vi "THz Time(SR830_VC)_Delay_LGS.vi"(1 "ESP300 Axis1":i8=1, 2 "ESP300 Address1":string="1", 4 "Lockin Address":string="12") -> ()   [LabVIEW 2010]
uses:
  <vilib>/Utility/file.llb/Write To Spreadsheet File (DBL).vi
panel:
  out "Boolean 2":bool
  in  "Position 3":sgl=3.4 format="%#.4f"
  in  "Set Position 2":bool
  out "error out":errorcluster
  out "Position 2":dbl[](array[numeric])=[2.395] format="%.6f"
  in  "error in":errorcluster
  out "Running":bool caption="Mercury_GCS_Configuration_Setup.vi is running"
  out "Conn. Axis":string[](array[string])=["1"]
  out "Identification":string="(c)2013 Physik Instrumente(PI) Karlsruhe, C-863.11,0,1.3.0.7"
  in  "SaveFile name":string="t"
  in  "Interdelay (ms)":dbl=10.0
  in  "pre delay(ms)":dbl=100.0
  out "Current deceleration":dbl=100.0
  in  "Acceleration":dbl
  out "Current acceleration":dbl=100.0
  in  "Set Acc":bool
  out "Current Velocity":dbl=25.0
  in  "Delay1 Stage":dbl
  in  "Set Velocity":bool
  in  "Reset Range":bool
  out "Boolean":bool
  out "MinValue":dbl format="%#.3p"
  out "MinPosition":dbl format="%#.3f"
  out "Lock-in Y-Channel":dbl=-7.0941e-11 format="%#.3p"
  out "Lock-in X-Channel":dbl=5.62071e-10 format="%#.3p"
  out "THz Time-domain Signal Wave":cluster{"x-axis":sgl[], "y-axis":dbl[]}(graph)={"x-axis"=[3.4, 3.395, 3.39, 3.385, 3.38, 3.375, 3.3700001, 3.365, 3.3600001, 3.355, 3.3500001, 3.345, 3.3400002, 3.335, 3.3300002, 3.325, 3.3200002, 3.315, 3.3100002, 3.305, 3.3000002, 3.295, 3.2900002, 3.285, 3.2800002, 3.275, 3.27, 3.265, 3.26, 3.255, 3.25, 3.2450001, 3.24, 3.2350001, 3.23, 3.2250001, 3.22, 3.2150002, 3.21, 3.2050002, 3.2, 3.1950002, 3.19, 3.1850002, 3.18, 3.1750002, 3.17, 3.1650002, 3.16, 3.1550002, 3.15, 3.1450002, 3.14, 3.135, 3.13, 3.125, 3.1200001, 3.115, 3.1100001, 3.105, 3.1000001, 3.095, 3.0900002, 3.085, 3.0800002, 3.075, 3.0700002, 3.065, 3.0600002, 3.055, 3.0500002, 3.045, 3.0400002, 3.035, 3.0300002, 3.025, 3.0200002, 3.015, 3.01, 3.005, 3.0, 2.9950001, 2.99, 2.9850001, 2.98, 2.9750001, 2.97, 2.9650002, 2.96, 2.9550002, 2.95, 2.9450002, 2.94, 2.9350002, 2.93, 2.9250002, 2.92, 2.9150002, 2.91, 2.9050002, 2.9, 2.8950002, 2.89, 2.885, 2.88, 2.875, 2.8700001, 2.865, 2.8600001, 2.855, 2.8500001, 2.845, 2.8400002, 2.835, 2.8300002, 2.825, 2.8200002, 2.815, 2.8100002, 2.805, 2.8000002, 2.795, 2.7900002, 2.785, 2.7800002, 2.775, 2.7700002, 2.765, 2.7600002, 2.755, 2.75, 2.7450001, 2.74, 2.7350001, 2.73, 2.7250001, 2.72, 2.7150002, 2.71, 2.7050002, 2.7, 2.6950002, 2.69, 2.6850002, 2.68, 2.6750002, 2.67, 2.6650002, 2.66, 2.6550002, 2.65, 2.6450002, 2.64, 2.6350002, 2.63, 2.625, 2.6200001, 2.615, 2.6100001, 2.605, 2.6000001, 2.595, 2.5900002, 2.585, 2.5800002, 2.575, 2.5700002, 2.565, 2.5600002, 2.555, 2.5500002, 2.545, 2.5400002, 2.535, 2.5300002, 2.525, 2.5200002, 2.515, 2.5100002, 2.505, 2.5, 2.4950001, 2.49, 2.4850001, 2.48, 2.4750001, 2.47, 2.4650002, 2.46, 2.4550002, 2.45, 2.4450002, 2.44, 2.4350002, 2.43, 2.4250002, 2.42, 2.4150002, 2.41, 2.4050002, 2.4, 2.3950002], "y-axis"=array[202 elements]}
  in  "Autosave Directory for Long-term Average Scan":path=path "D:/Soon/140901_delay_test/2_VC_delay_ESP_-2.35/1_VC_delay"
  out "Phase":cluster{"f0":dbl, "df":dbl, "magnitude":dbl[]}(graph)={"f0"=0.0, "df"=0.14851486070616432, "magnitude"=[3.141592653589793, -1.1082186029585688, 2.1245945726281503, -0.5802126962218755, 2.9522431871923738, 0.25355132108658424, -2.5001587400129117, 1.0450360548561866, -1.6833529420673685, 1.9054335161918228, -0.7535788037728205, 2.8437560114605995, 0.1867891479959547, -2.5687719161866958, 1.0293610676943812, -1.7670984731304367, 1.7396136198319216, -0.989399029539729, 2.5333749473756697, 0.8404425122915157, -3.0418476408700195, 1.801491493426078, 1.2291977401939342, 2.193306480389313, 1.1536290801184514, 2.257021637212434, 1.4812870523644348, 2.188959750025471, 1.966995842051201, 1.8991000587928113, 2.316846473675966, 1.7957148476473666, 2.343784775169297, 2.055723593650246, 1.8995404855444666, 2.3374703620389807, 1.7334801576564551, 2.5115455204750092, 1.9597467730439078, 2.2954790599099035, 2.198181356679205, 2.1422497310116677, 2.228848712078954, 2.3604901133382894, 1.9776993845037527, 2.602909416876564, 2.0799347375491797, 2.4419998834544696, 2.3534588247198736, 2.2439655455562337, 2.367780240538884, 2.4173118073649276, 2.13794690411644, 2.6001847828499938, 2.2538070428436865, 2.4392433056261886, 2.5322980937687722, 2.33220876018927, 2.5581206126688922, 2.4920111361083035, 2.365959844925607, 2.6396344462612515, 2.387346853088604, 2.663819735565773, 2.503292776172557, 2.6066427525464575, 2.596199386556665, 2.5917147401712675, 2.5966251179974464, 2.6741740931066458, 2.575163618331821, 2.758796254024769, 2.606630146141833, 2.698588779947026, 2.779755754618168, 2.636241327225838, 2.859969608313545, 2.68829051279584, 2.7969939565985547, 2.795740014252736, 2.7620236189146024, 2.857190149539915, 2.8576368807511114, 2.7988186860636706, 2.9527385937994426, 2.8126212545415386, 2.9271634690601185, 2.96078760907565, 2.7401621755492296, -3.0621438857467163, 2.5801858239187037, -2.741093203572613, 2.771636401079869, -2.8921243601658513, -3.091948951572802, 1.9572111607568423, -2.7375815827125485, 2.554987619803606, -2.850283932292324, 3.0341936848447073, 3.139143526249259]}
  out "elapsed time":string=" 0 h  12 m  48 s"
  in  "OK Button":bool
  out "Data Type":string="outp ? 1"
  in  "Enum":enum16{"X", "Y", "Abs"}(ring)
  out "MaxValue":dbl format="%#.3p"
  out "MaxPosition":dbl format="%#.3f"
  in  "Position":sgl format="%#.4f"
  in  "Find Max":bool
  in  "Set Position":bool
  in  "Save Data":bool
  in  "SCAN":bool
  in  "Exit Program":bool
  out "Amplitude":cluster{"f0":dbl, "df":dbl, "magnitude":dbl[]}(graph)={"f0"=0.0, "df"=0.14851486070616432, "magnitude"=[3.52573264851484e-11, 8.389855621430922e-10, 2.225761799960767e-09, 3.4042126658161336e-09, 4.230842896022254e-09, 4.467306313802578e-09, 4.228754619739681e-09, 3.6175759039566052e-09, 2.7932538533113405e-09, 2.0909677390642694e-09, 1.4830038497464771e-09, 1.0735909873360868e-09, 7.513836201453385e-10, 5.085801170819804e-10, 3.409708772444367e-10, 2.0157630953836574e-10, 1.3092497815900202e-10, 5.049635088240611e-11, 3.21982450563289e-11, 1.6834701069452993e-11, 7.165882992001707e-12, 1.3534244019293799e-11, 2.2560794068677396e-12, 1.0955642605171567e-11, 3.936119948051029e-12, 9.190533457493373e-12, 4.4193088993100694e-12, 6.762265647261314e-12, 4.993312878347624e-12, 5.062736813562155e-12, 5.24252743088094e-12, 5.787564208573698e-12, 3.5338798468168525e-12, 6.289625941575823e-12, 2.9009219878310403e-12, 5.735399147740872e-12, 4.098798711026944e-12, 4.0941543980206186e-12, 5.005680034820198e-12, 2.9952585898831173e-12, 4.635819232904141e-12, 3.483558839132468e-12, 3.5438954539821336e-12, 4.019219618061033e-12, 3.530627852632409e-12, 3.4790764329431817e-12, 4.215077525071282e-12, 2.6292492576384014e-12, 3.696721717997553e-12, 3.400423534031585e-12, 2.5887642494668405e-12, 3.943756030791582e-12, 2.5289746794441754e-12, 3.401204539630353e-12, 3.10293276186898e-12, 2.786775807858238e-12, 2.9186601113132677e-12, 3.284595365146064e-12, 2.271033822874899e-12, 3.5054000253471667e-12, 2.2657565242544363e-12, 3.112172318680258e-12, 2.6330104473143568e-12, 2.7634443891954928e-12, 2.7484453359122282e-12, 2.592035676554931e-12, 2.5633028950781254e-12, 2.6521106649509693e-12, 2.360345428093699e-12, 2.7497689895804224e-12, 2.3635944544452143e-12, 2.5866385290965327e-12, 2.5442012769231896e-12, 2.298983787328914e-12, 2.624194910906667e-12, 2.384593975973384e-12, 2.3523429224266368e-12, 2.5577359065613025e-12, 2.221370415250699e-12, 2.4629634177599407e-12, 2.3284037072725584e-12, 2.2392891386041413e-12, 2.4830764922560122e-12, 2.1850697748689936e-12, 2.3325327936824436e-12, 2.4734800041535514e-12, 2.041958899932065e-12, 2.6672550572923e-12, 1.847654298403158e-12, 2.668652435775197e-12, 2.456539312232025e-12, 1.9162881391774236e-12, 3.5876527691091694e-12, 5.308809354301319e-13, 4.197872609875915e-12, 1.5590595736913964e-12, 3.349567160539913e-12, 2.5611964195912033e-12, 2.0676305856675026e-12, 2.350754443680646e-12, 2.2948601507955558e-12]}
  in  "Short term \nAverage#":i8=2
  out "Numeric 2":i8=15
  in  "Long term Average#":dbl=16.0
  in  "Step":sgl=0.005 min=0 max=10000 format="%.3f"
  in  "End Postion":sgl=2.4 min=-400 max=400 format="%#.3f"
  in  "Start Position":sgl=3.4 min=-400 max=400 format="%#.3f"
  # "This Program Run First (1) and then Run the Approach Program (2)"
  # "THz Experiment"
  # "``"
  # "Auto-offset"
  # "Input Data"
  # "Delay Line (VC)"
  # "Point Avg"
  # "Long Avg"
  # "Turn Number"
  # "mm"
  # "mm"
  # "MAX"
  # "MIN"
  # "other step\nposition"
  # "stage \nposition"
  # "stage \nposition"
  # "value"
  # "value"
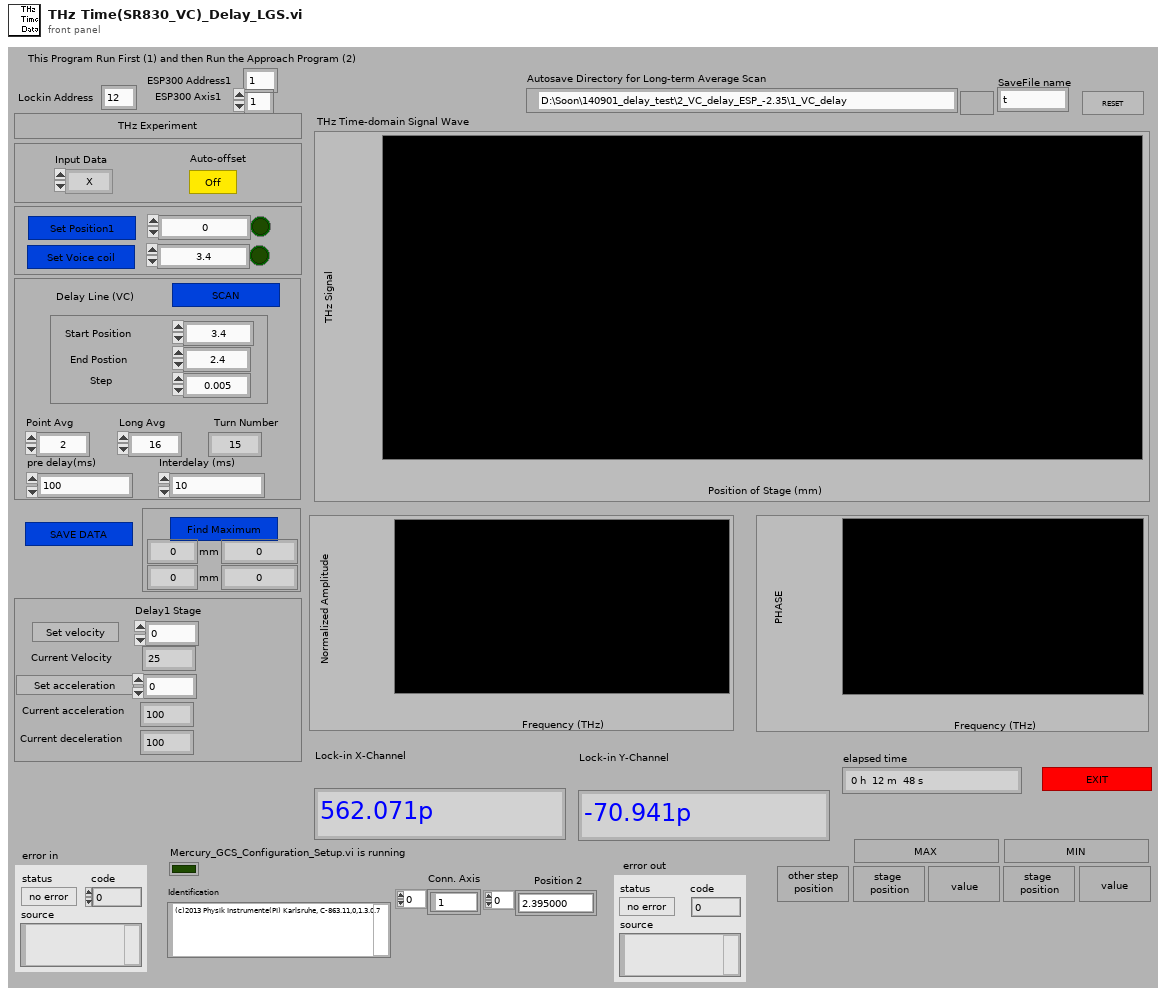
[diagram p1: front panel]
types:
  T1 = cluster{"System no.":i32, "error out":errorcluster}
  T2 = cluster{"Step Number":i32, "Step":sgl, "Start Position":sgl, "Time-out":i32, "Lockin Address":string, "Short term \nAverage#":i8, "System no.":i32, "error out":errorcluster, "Value":string, "pre delay(ms)":dbl, "Interdelay (ms)":dbl, "Autosave Directory for Long-term Average Scan":path}
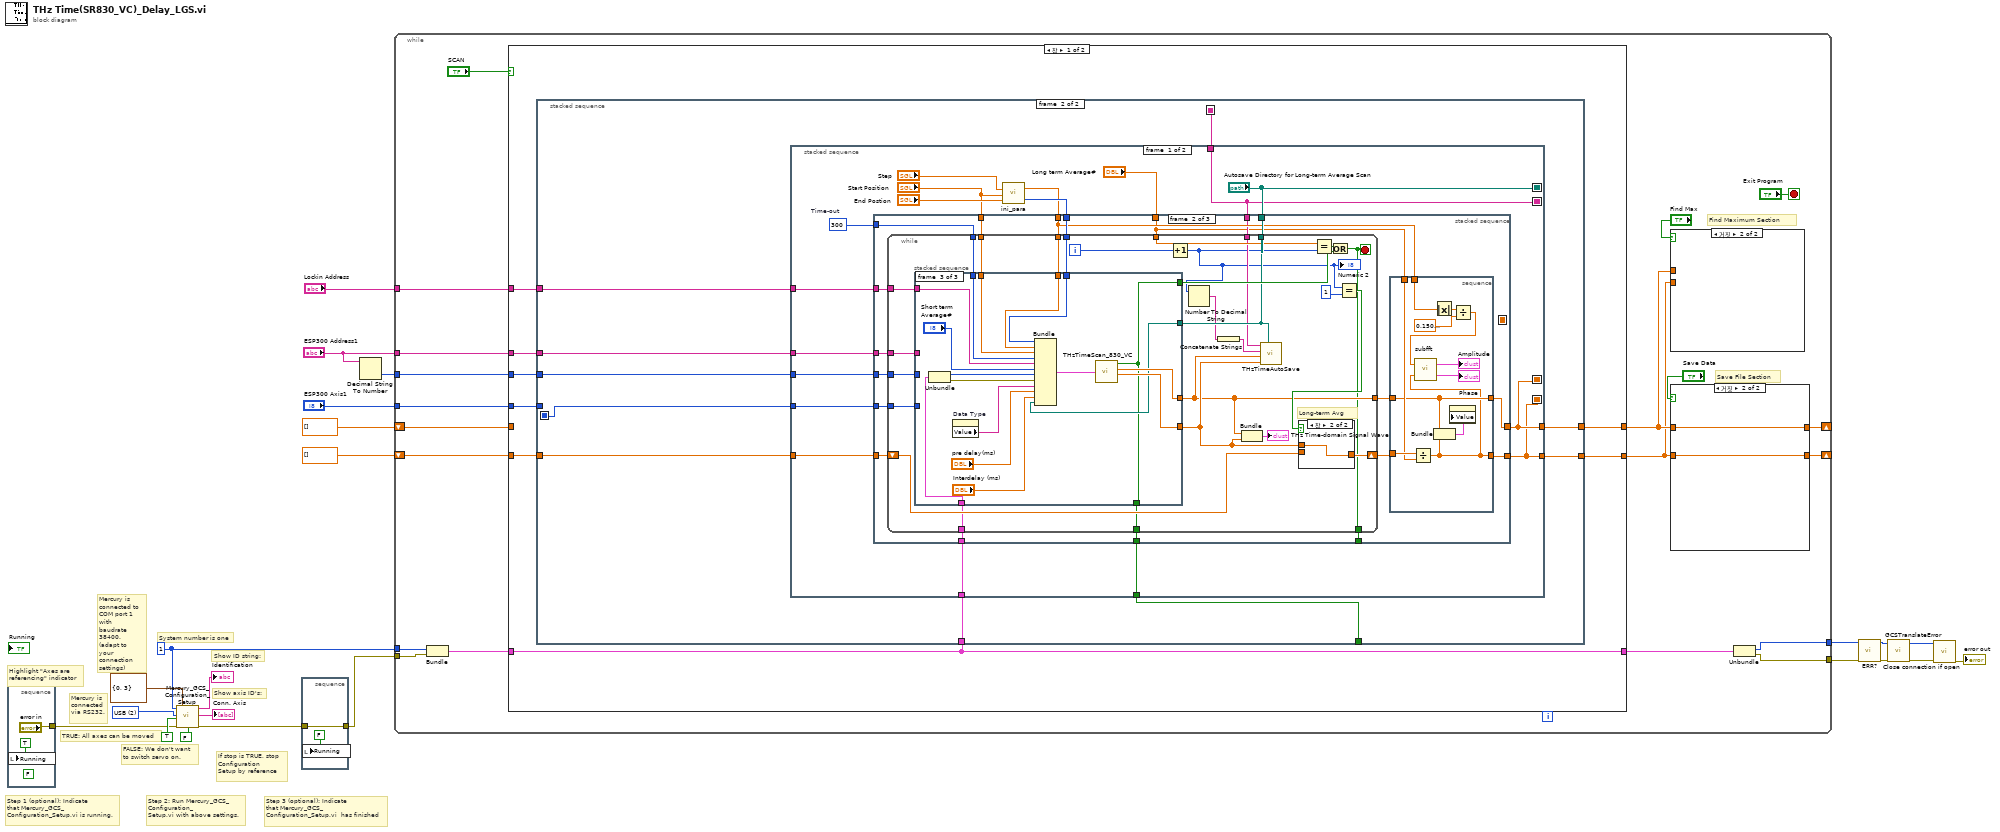
[diagram p0: block diagram]
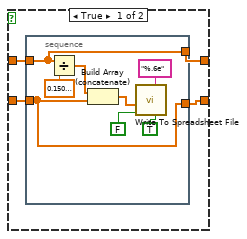
[diagram p2: hidden frame]
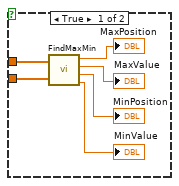
[diagram p3: hidden frame]
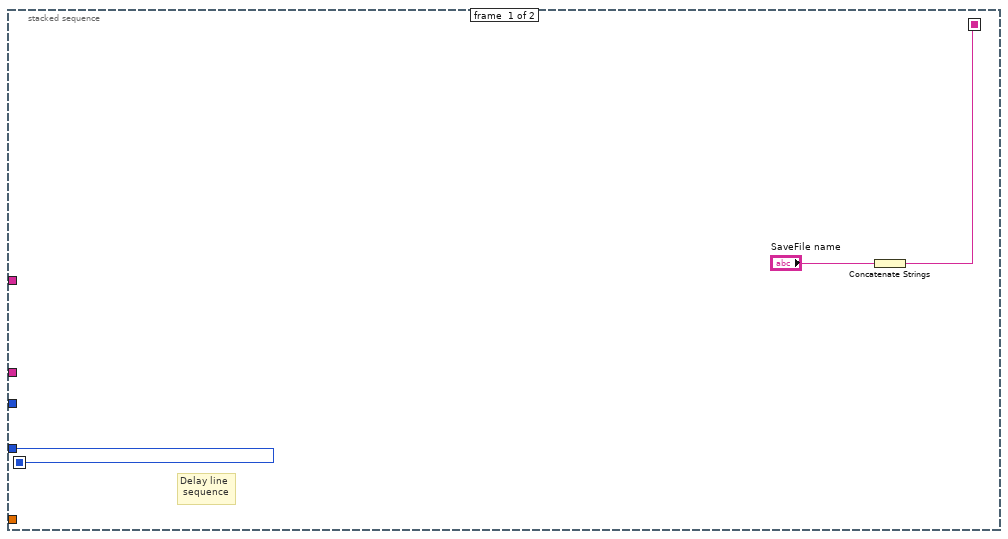
[diagram p4: hidden frame]
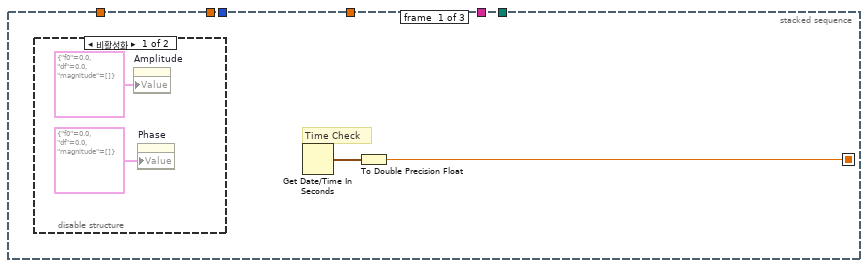
[diagram p5: hidden frame]
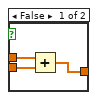
[diagram p7: hidden frame]
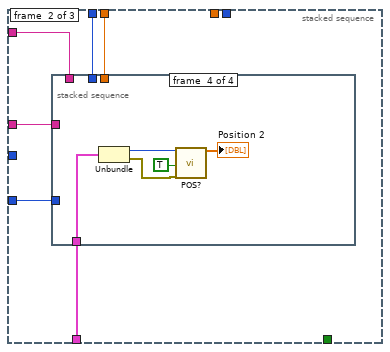
[diagram p9: hidden frame]
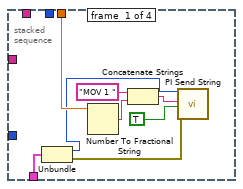
[diagram p10: hidden frame]
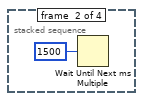
[diagram p11: hidden frame]
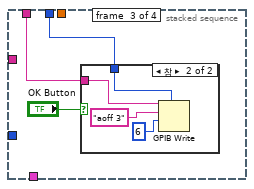
[diagram p12: hidden frame]
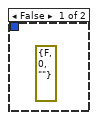
[diagram p13: hidden frame]
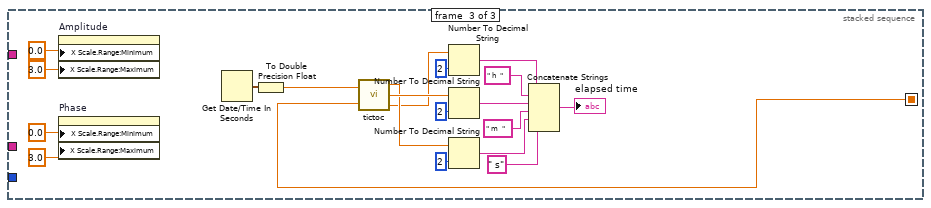
[diagram p14: hidden frame]
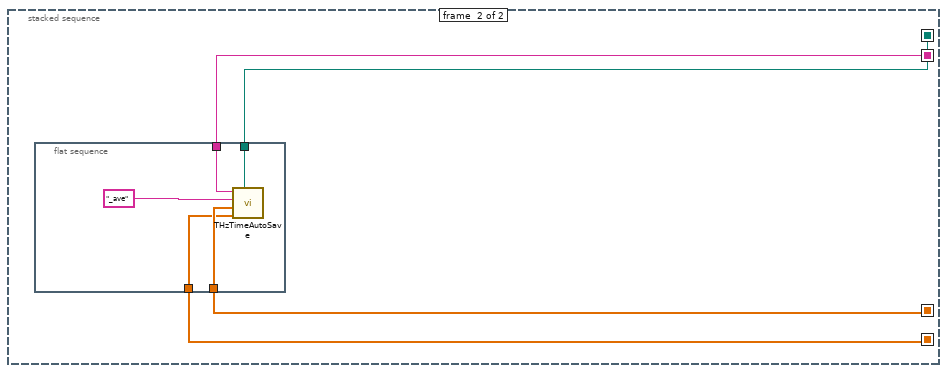
[diagram p15: hidden frame]
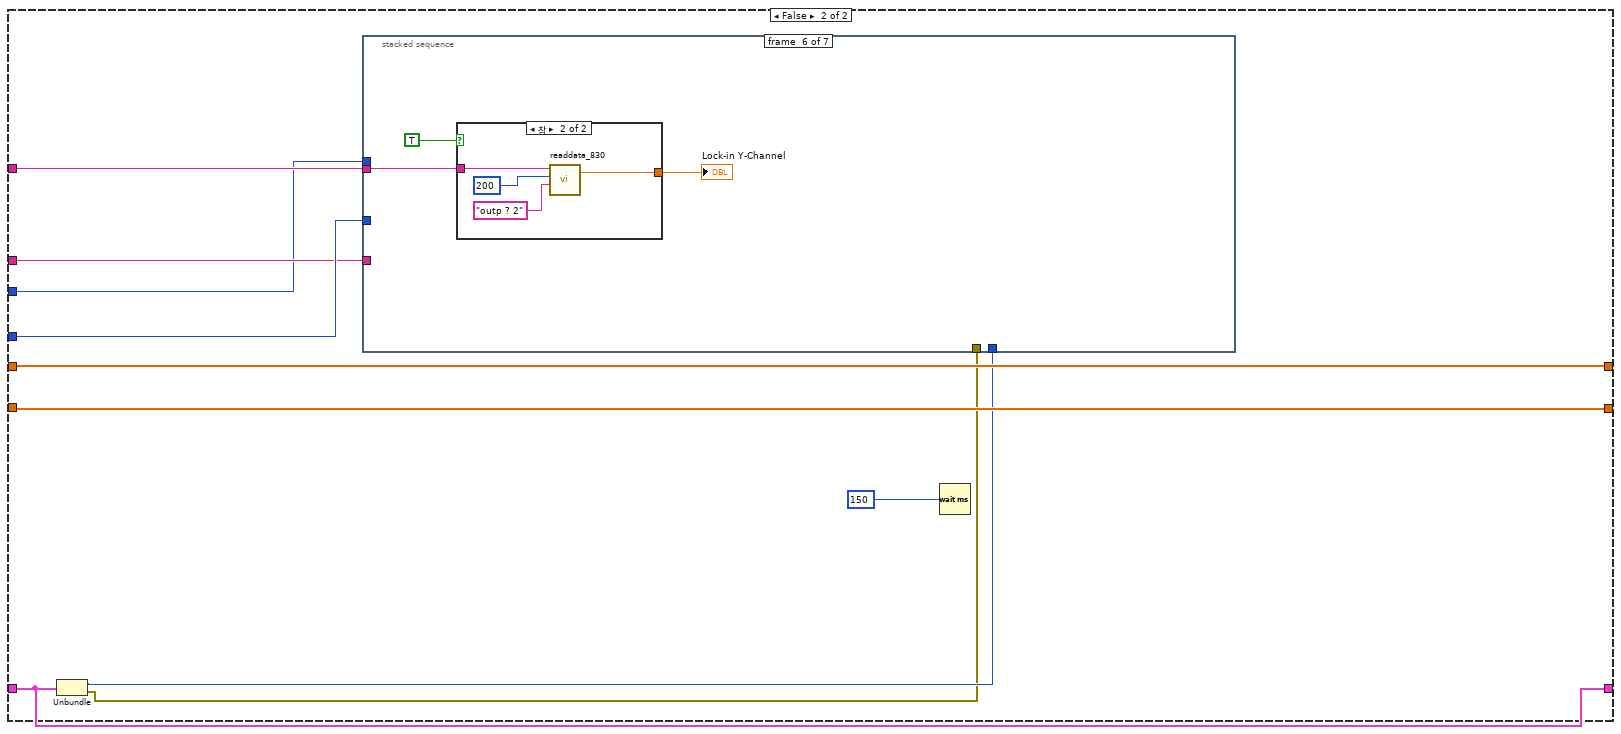
[diagram p16: hidden frame]
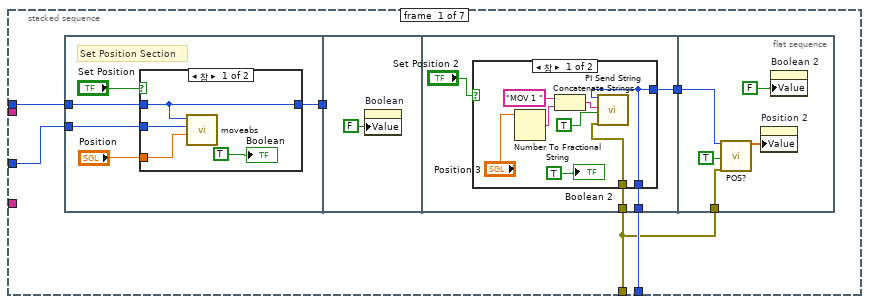
[diagram p17: hidden frame]
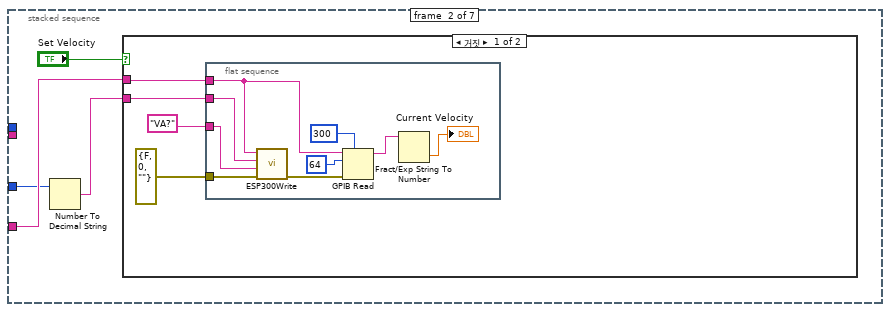
[diagram p20: hidden frame]
diagram:
  w8 = u16 2 items=["RS232", "RS232 DaisyChain", "USB", "USB_DaisyChain"] ("Interface")
  w7 = 1 ("System no.")
  # "Mercury is\nconnected\nvia RS232."
  # "If stop is TRUE, stop \nConfiguration\nSetup by reference"
  # "Mercury is\nconnected to\nCOM port 1\nwith baudrate\n38400.\n(adapt to your\nconnection\nsettings)"
  # "Step 3 (optional): Indicate\nthat Mercury_GCS_\nConfiguration_Setup.vi  has finished"
  # "Step 2: Run Mercury_GCS_\nConfiguration_\nSetup.vi with above settings."
  # "Step 1 (optional): Indicate\nthat Mercury_GCS_\nConfiguration_Setup.vi is running."
  # "Highlight \"Axes are\nreferencing\" indicator"
  # "Show axis ID's:"
  # "Show ID string:"
  # "FALSE: We don't want\nto switch servo on."
  # "TRUE: All axes can be moved"
  # "System number is one"
  n1 = stacked-sequence {
    tunnel: ["error in"] -> w11
    frame #0 {
      (unwired) FALSE ("stop")
      n2 = local write "Running"(TRUE ("Running")) -> ()
    }
  }
  n3 = call "Mercury_GCS_Configuration_Setup.vi"("System no."=w7, "Interface"=w8, "All axes?"=TRUE, "error in"=w11, "RS232 settings"=cluster{"RS232 Portnumber":i32, "Baudrate":u16} {"RS232 Portnumber"=0, "Baudrate"=3}, "Switch servo on?"=FALSE ("Use dialog to define\nconnected stages?")) -> ("Identification"=→"Identification":string, "Conn. \nAxes"=→"Conn. Axis":string[], "error out"=w12:errorcluster)  [unwired: 7 in, 4 out]
  n4 = stacked-sequence {
    tunnel: w12 -> [w25]
    tunnel: [w25] -> w6
    frame #0 {
      n5 = local write "Running"(FALSE ("Running")) -> ()
    }
  }
  n6 = Decimal String To Number(string="ESP300 Address1") -> (number=w16:i32)  [unwired: 2 in, 1 out]
  n7 = while {
    tunnel: "ESP300 Axis1" -> [w41]
    tunnel: "Lockin Address" -> [w33]
    shift-right: [w38] -> _
    shift-left: sgl[] [] -> [w40]
    shift-right: [w37] -> _
    shift-left: dbl[] [] -> [w39]
    tunnel: "ESP300 Address1" -> [w34]
    tunnel: w16 -> [w32]
    tunnel: w7 -> [w31]
    tunnel: w6 -> [w30]
    tunnel: [w27] -> w2
    tunnel: [w26] -> w1
    stop <- "Exit Program" stop-if-true
    # "Save File Section"
    # "Find Maximum Section"
    n8 = Bundle("System no."=w31, "error out"=w30) -> (w29:T1)  [unwired: 1 in]
    n9 = case shown="참" "SCAN" {
      tunnel: w41 -> [w73 w252]
      tunnel: [w72 w249] -> w36
      tunnel: [w71 w248] -> w35
      tunnel: w40 -> [_ w249]
      tunnel: w39 -> [w70 w248]
      tunnel: w34 -> [w69 w250]
      tunnel: w33 -> [w68 w247]
      tunnel: w32 -> [w67 w246]
      tunnel: w29 -> [w66 w243]
      tunnel: [w66 w243] -> w28
      frame True {
        n10 = stacked-sequence {
          seq-local: [w76 _] -> [_ w79]
          seq-local: [w74 _] -> [_ w80]
          tunnel: w73 -> [w76 _]
          tunnel: [_ w86] -> w72
          tunnel: [_ w85] -> w71
          tunnel: w70 -> [_ w84]
          tunnel: w69 -> [_ w83]
          tunnel: w68 -> [_ w82]
          tunnel: w67 -> [_ w81]
          tunnel: [_ w77] -> _
          tunnel: w66 -> [_ w78]
          frame #0 {
            # "Delay line\n sequence"
            n11 = Concatenate Strings("SaveFile name") -> (w74:string)
          }
          frame #1 {
            n12 = stacked-sequence {
              seq-local: [w94 _] -> [_ w235]
              seq-local: [w93 _] -> [_ w234]
              seq-local: ["Autosave Directory for Long-term Average Scan" _] -> [_ w236]
              seq-local: [w89 _] -> [_ w237]
              tunnel: w79 -> [w104 _]
              tunnel: [w94 _] -> w86
              tunnel: [w93 _] -> w85
              tunnel: w84 -> [w97 _]
              tunnel: w83 -> [w96 _]
              tunnel: [w95 _] -> w77
              tunnel: w82 -> [w91 _]
              tunnel: w81 -> [w90 _]
              tunnel: w80 -> [w89 _]
              tunnel: w78 -> [w87 _]
              frame #0 {
                w103 = 300  # Time-out
                n13 = call "ini_para.vi"("End Position"="End Postion", "Start Position"="Start Position", "Step"="Step") -> ("Step Number"=w100:i32, "Step"=w99:sgl)
                n14 = stacked-sequence {
                  seq-local: [w105 _ _] -> [_ _ w214]
                  tunnel: w103 -> [_ w127 _]
                  tunnel: "Long term Average#" -> [_ w110 _]
                  tunnel: w104 -> [_ w126 _]
                  tunnel: w100 -> [_ w124 _]
                  tunnel: w99 -> [_ w122 _]
                  tunnel: "Start Position" -> [_ w125 _]
                  tunnel: "Autosave Directory for Long-term Average Scan" -> [_ w123 _]
                  tunnel: [_ w113 _] -> w94
                  tunnel: [_ w121 _] -> w93
                  tunnel: w97 -> [_ w119 _]
                  tunnel: w96 -> [_ w120 _]
                  tunnel: w89 -> [_ w118 _]
                  tunnel: [_ w117 _] -> w95
                  tunnel: w91 -> [_ w116 _]
                  tunnel: w90 -> [_ w115 _]
                  tunnel: [_ w111 _] -> _
                  tunnel: w87 -> [_ w109 _]
                  frame #0 {
                    # "Time Check"
                    n15 = disable-structure shown="비활성화" {
                      frame Disabled {
                        n16 = property on="Amplitude" class="WFGraph (엄격한)"("Value"=cluster{"f0":dbl, "df":dbl, "magnitude":dbl[]} {"f0"=0.0, "df"=0.0, "magnitude"=[]} ("Spectrum")) -> ()  [unwired: 2 in, 2 out]
                        n17 = property on="Phase" class="WFGraph (엄격한)"("Value"=cluster{"f0":dbl, "df":dbl, "magnitude":dbl[]} {"f0"=0.0, "df"=0.0, "magnitude"=[]} ("Spectrum")) -> ()  [unwired: 2 in, 2 out]
                      }
                      frame Enabled {
                      }
                    }
                    n18 = Get Date/Time In Seconds() -> (seconds since 1Jan1904=w106:timestamp)
                    n19 = To Double Precision Float(number=w106) -> (double precision float=w105:dbl)
                  }
                  frame #1 {
                    n20 = while {
                      tunnel: w110 -> [w164]
                      tunnel: w127 -> [w165]
                      tunnel: w126 -> [w161]
                      tunnel: w125 -> [w160]
                      tunnel: w122 -> [w159]
                      tunnel: w124 -> [w158]
                      tunnel: w123 -> [w153]
                      shift-right: [w144] -> w112
                      shift-left: w119 -> [w156]
                      tunnel: [w146] -> w114
                      tunnel: w120 -> [w155]
                      tunnel: w118 -> [w152]
                      tunnel: [w154] -> w117
                      tunnel: w116 -> [w149]
                      tunnel: w115 -> [w148]
                      tunnel: [w143] -> w111
                      tunnel: w109 -> [w141]
                      i -> [w140]
                      stop <- w143 stop-if-true
                      # "Long-term Avg"
                      n21 = stacked-sequence {
                        tunnel: w165 -> [_ w175 w212]
                        tunnel: [_ _ w204] -> w162
                        tunnel: w161 -> [_ w174 _]
                        tunnel: w160 -> [_ w173 w200]
                        tunnel: w159 -> [_ _ w201]
                        tunnel: w158 -> [_ _ w213]
                        tunnel: [_ _ w209] -> w146
                        tunnel: [_ _ w208] -> w150
                        tunnel: w155 -> [_ w172 _]
                        tunnel: w153 -> [_ _ w205]
                        tunnel: [_ _ w204] -> w154
                        tunnel: w149 -> [_ w171 w203]
                        tunnel: w148 -> [_ _ _]
                        tunnel: w141 -> [_ w170 w199]
                        frame #0 {
                        }
                        frame #1 {
                          n22 = stacked-sequence {
                            tunnel: w175 -> [_ _ w186 _]
                            tunnel: w174 -> [_ _ _ _]
                            tunnel: w173 -> [w179 _ _ _]
                            tunnel: w172 -> [_ _ _ _]
                            tunnel: w171 -> [_ _ w185 _]
                            tunnel: w170 -> [w178 _ _ w194]
                            frame #0 {
                              n23 = Unbundle(w178) -> ("System no."=w176:i32, "error out"=w177:errorcluster)
                              n24 = Number To Fractional String(number=w179) -> (F-format string=w180:string)  [unwired: 3 in]
                              n25 = Concatenate Strings("MOV 1 ", w180) -> (w183:string)
                              n26 = call "PI Send String.vi"("System no."=w176, "String to send"=w183, "Attach termination char.?"=TRUE ("Attach Linefeed?"), "error in"=w177) -> ()  [unwired: 15 in, 1 out]
                            }
                            frame #1 {
                              n27 = Wait Until Next ms Multiple(millisecond multiple=1500) -> ()  [unwired: 1 out]
                            }
                            frame #2 {
                              n28 = case shown="참" "OK Button" {
                                tunnel: w186 -> [_ w190]
                                tunnel: w185 -> [_ w188]
                                frame False {
                                (unwired) errorcluster {"status"=FALSE, "code"=0, "source"=""} ("error in")
                                }
                                frame True {
                                n29 = GPIB Write(0:w188, 1:"aoff 3" ("data"), 2:i16 6 ("mode (0)"), 4:w190) -> ()  [unwired: 1 in, 2 out]
                                }
                              }
                            }
                            frame #3 {
                              n30 = Unbundle(w194) -> ("System no."=w193:i32, "error out"=w192:errorcluster)
                              n31 = call "POS?.vi"("System no."=w193, "All axes?"=TRUE, "error in"=w192) -> ("Position"=→"Position 2":dbl[])  [unwired: 15 in, 1 out]
                            }
                          }
                        }
                        frame #2 {
                          n32 = Unbundle(w199) -> ("System no."=w198:i32, "error out"=w197:errorcluster)
                          n33 = property on="Data Type" class="Str"() -> ("Value"=w210:string)  [unwired: 2 in, 2 out]
                          n34 = Bundle("Step Number"=w213, "Step"=w201, "Start Position"=w200, "Time-out"=w212, "Lockin Address"=w203, "Short term \nAverage#"="Short term \nAverage#", "System no."=w198, "error out"=w197, "Value"=w210, "pre delay(ms)"="pre delay(ms)", "Interdelay (ms)"="Interdelay (ms)", "Autosave Directory for Long-term Average Scan"=w205) -> (w202:T2)  [unwired: 1 in]
                          n35 = call "THzTimeScan_830_VC.vi"("input"=w202) -> ("loop stop"=w204:bool, "x-axis"=w209:sgl[], "y-axis"=w208:dbl[])  [unwired: 1 in]
                        }
                      }
                      n36 = Increment(x=w140) -> (x+1=w139:i32)
                      "Numeric 2" <- w139
                      n37 = Number To Decimal String(number=w139) -> (decimal integer string=w142:string)  [unwired: 1 in]
                      n38 = Concatenate Strings(w142) -> (w151:string)
                      n39 = Bundle("x-axis"=w146, "y-axis"=w150) -> (→"THz Time-domain Signal Wave":cluster{"x-axis":sgl[], "y-axis":dbl[]})  [unwired: 1 in]
                      n40 = call "THzTimeAutoSave.vi"("Autosave Directory for Long-term Average Scan"=w153, "y-axis"=w150, "x-axis"=w146, "String"=w151, "SaveFile name"=w152) -> ()  [unwired: 5 in]
                      n41 = Equal?(x=w164, y=w139) -> (x = y?=w163:bool)
                      n42 = Or(x=w163, y=w162) -> (x .or. y?=w143:bool)
                      n43 = Equal?(x=w139, y=1) -> (x = y?=w147:bool)
                      n44 = case shown="참" w147 {
                        tunnel: w156 -> [w167 _]
                        tunnel: w150 -> [w168 w169]
                        tunnel: [w166 w169] -> w144
                        frame False {
                          n45 = Add(x=w168, y=w167) -> (x+y=w166:dbl[])
                        }
                        frame True {
                        }
                      }
                    }
                    n46 = stacked-sequence {
                      tunnel: w122 -> [w133]
                      tunnel: w114 -> [w129]
                      tunnel: w112 -> [w131]
                      tunnel: [w128] -> w121
                      tunnel: w110 -> [w130]
                      tunnel: [w129] -> w113
                      frame #0 {
                        n47 = Divide(x=w131, y=w130) -> (x/y=w128:dbl[])
                        n48 = Absolute Value(x=w133) -> (abs(x)=w134:sgl)
                        n49 = Bundle("x-axis"=w129, w128) -> (w138:cluster{"x-axis":sgl[], dbl[]})  [unwired: 1 in]
                        n50 = property on="THz Time-domain Signal Wave" class="XYGraph (엄격한)"("Value"=w138) -> ()  [unwired: 2 in, 2 out]
                        n51 = Divide(x=w134, y=sgl 0.15) -> (x/y=w132:sgl)
                        n52 = call "subfft.vi"("y-signal"=w128, "time step"=w132) -> ("Phase"=→"Phase":cluster{"f0":dbl, "df":dbl, "real part":dbl[]}, "Amplitude"=→"Amplitude":cluster{"f0":dbl, "df":dbl, "real part":dbl[]})
                      }
                    }
                  }
                  frame #2 {
                    n53 = property on="Amplitude" class="WFGraph (엄격한)"("X Scale.Range:Minimum"=0.0 ("X Scale.Range:Maximum"), "X Scale.Range:Maximum"=3.0) -> ()  [unwired: 2 in, 2 out]
                    n54 = property on="Phase" class="WFGraph (엄격한)"("X Scale.Range:Minimum"=0.0, "X Scale.Range:Maximum"=3.0) -> ()  [unwired: 2 in, 2 out]
                    n55 = Get Date/Time In Seconds() -> (seconds since 1Jan1904=w219:timestamp)
                    n56 = To Double Precision Float(number=w219) -> (double precision float=w218:dbl)
                    n57 = call "tictoc.vi"("Value"=w218, "Value 2"=w214) -> ("sec"=w216:dbl, "min"=w217:dbl, "hour"=w215:dbl)
                    n58 = Number To Decimal String(number=w215, width (-)=i16 2) -> (decimal integer string=w224:string)
                    n59 = Number To Decimal String(number=w217, width (-)=i16 2) -> (decimal integer string=w230:string)
                    n60 = Number To Decimal String(number=w216, width (-)=i16 2) -> (decimal integer string=w229:string)
                    n61 = Concatenate Strings(w224, " h  " ("Substring"), w230, " m  " ("Substring"), w229, " s" ("Substring")) -> (→"elapsed time":string)
                  }
                }
              }
              frame #1 {
                n62 = flat-sequence {
                  tunnel: w236 -> [w242]
                  tunnel: w237 -> [w241]
                  tunnel: w235 -> [w240]
                  tunnel: w234 -> [w239]
                  frame #0 {
                    n63 = call "THzTimeAutoSave.vi"("Autosave Directory for Long-term Average Scan"=w242, "y-axis"=w239, "x-axis"=w240, "String"="_ave" ("string"), "SaveFile name"=w241) -> ()  [unwired: 5 in]
                  }
                }
              }
            }
          }
        }
      }
      frame False {
        n64 = Unbundle(w243) -> ("System no."=w245:i32, "error out"=w244:errorcluster)
        n65 = stacked-sequence {
          tunnel: w252 -> [w258 w289 w318 _ _ _ _]
          tunnel: w250 -> [_ w290 w319 _ _ _ _]
          tunnel: w247 -> [_ _ _ _ w376 w385 _]
          tunnel: w246 -> [w257 _ _ _ _ _ _]
          tunnel: w245 -> [w255 _ _ _ _ _ _]
          tunnel: w244 -> [w253 _ _ _ _ _ _]
          frame #0 {
            n66 = flat-sequence {
              tunnel: w258 -> [w263]
              tunnel: w257 -> [w260]
              tunnel: [w259] -> w256
              tunnel: w256 -> [_]
              tunnel: w255 -> [w272]
              tunnel: w253 -> [w271]
              tunnel: [w270] -> w254
              tunnel: w254 -> [w285]
              tunnel: w253 -> [w284]
              frame #0 {
                # "Set Position Section"
                n67 = case shown="참" "Set Position" {
                  tunnel: "Position" -> [w267 _]
                  tunnel: w263 -> [w266 _]
                  tunnel: w260 -> [w264 w268]
                  tunnel: [w264 w268] -> w259
                  frame True {
                    n68 = call "moveabs.vi"("SetPosition"=w267, "EXP300 -3A Axis"=w266, "ESP300 -3A Add."=w264) -> ()  [unwired: 2 in]
                    "Boolean" <- TRUE
                  }
                  frame False {
                  }
                }
              }
              frame #1 {
                n69 = property on="Boolean" class="Bool (엄격한)"("Value"=FALSE ("Boolean")) -> ()  [unwired: 2 in, 2 out]
              }
              frame #2 {
                n70 = case shown="참" "Set Position 2" {
                  tunnel: w272 -> [w274 w282]
                  tunnel: w271 -> [w275 _]
                  tunnel: [w274 w282] -> w270
                  frame True {
                    n71 = Number To Fractional String(number="Position 3") -> (F-format string=w277:string)  [unwired: 3 in]
                    n72 = Concatenate Strings("MOV 1 ", w277) -> (w280:string)
                    n73 = call "PI Send String.vi"("System no."=w274, "String to send"=w280, "Attach termination char.?"=TRUE ("Attach Linefeed?"), "error in"=w275) -> ()  [unwired: 15 in, 1 out]
                    "Boolean 2" <- TRUE
                  }
                  frame False {
                  }
                }
              }
              frame #3 {
                n74 = call "POS?.vi"("System no."=w285, "All axes?"=TRUE, "error in"=w284) -> ("Position"=w287:dbl[])  [unwired: 15 in, 1 out]
                n75 = property on="Position 2" class="Arr (엄격한)"("Value"=w287) -> ()  [unwired: 2 in, 2 out]
                n76 = property on="Boolean 2" class="Bool (엄격한)"("Value"=FALSE ("Boolean")) -> ()  [unwired: 2 in, 2 out]
              }
            }
          }
          frame #1 {
            n77 = Number To Decimal String(number=w289) -> (decimal integer string=w288:string)  [unwired: 1 in]
            n78 = case shown="거짓" "Set Velocity" {
              tunnel: w290 -> [w292 w308]
              tunnel: w288 -> [w295 w309]
              frame False {
                n79 = flat-sequence {
                  tunnel: w295 -> [w304]
                  tunnel: errorcluster {"status"=FALSE, "code"=0, "source"=""} ("error in (no error)") -> [w297]
                  tunnel: "VA?" ("Command") -> [w298]
                  tunnel: w292 -> [w296]
                  frame #0 {
                    n80 = call "ESP300Write.vi"("error in (no error)"=w297, "Command"=w298, "ESP300 Axis"=w304, "ESP300 Address"=w296) -> ("error out"=w299:errorcluster)  [unwired: 3 in]
                    n81 = GPIB Read(0:w296, 1:64 ("byte count"), 3:w299, 4:300 ("timeout ms (488.2 global)")) -> (5:w303:string)  [unwired: 1 in, 2 out]
                    n82 = Fract/Exp String To Number(string=w303) -> (number=→"Current Velocity":dbl)  [unwired: 3 in, 1 out]
                  }
                }
              }
              frame True {
                n83 = flat-sequence {
                  tunnel: w309 -> [w317]
                  tunnel: w308 -> [w312]
                  tunnel: [w312] -> w307
                  tunnel: errorcluster {"status"=FALSE, "code"=0, "source"=""} ("error in (no error)") -> [w311]
                  tunnel: [w310] -> w305
                  tunnel: w307 -> [_]
                  tunnel: w305 -> [_]
                  frame #0 {
                    n84 = Number To Fractional String(number="Delay1 Stage") -> (F-format string=w315:string)  [unwired: 3 in]
                    n85 = Concatenate Strings("VA" ("string"), w315) -> (w313:string)
                    n86 = call "ESP300Write.vi"("error in (no error)"=w311, "Command"=w313, "ESP300 Axis"=w317, "ESP300 Address"=w312) -> ("error out"=w310:errorcluster)  [unwired: 3 in]
                  }
                  frame #1 {
                  }
                }
              }
            }
          }
          frame #2 {
            n87 = Number To Decimal String(number=w318) -> (decimal integer string=w320:string)  [unwired: 1 in]
            n88 = case shown="참" "Set Acc" {
              tunnel: w319 -> [w322 w347]
              tunnel: w320 -> [w323 w348]
              frame False {
                n89 = stacked-sequence {
                  tunnel: w323 -> [w325 w335]
                  tunnel: w322 -> [w324 w336]
                  frame #0 {
                    n90 = flat-sequence {
                      tunnel: w325 -> [w334]
                      tunnel: w324 -> [w327]
                      frame #0 {
                        n91 = call "ESP300Write.vi"("error in (no error)"=errorcluster {"status"=FALSE, "code"=0, "source"=""}, "Command"="AC?", "ESP300 Axis"=w334, "ESP300 Address"=w327) -> ("error out"=w328:errorcluster)  [unwired: 3 in]
                        n92 = GPIB Read(0:w327, 1:64 ("byte count"), 3:w328, 4:300 ("timeout ms (488.2 global)")) -> (5:w332:string)  [unwired: 1 in, 2 out]
                        n93 = Fract/Exp String To Number(string=w332) -> (number=→"Current acceleration":dbl)  [unwired: 3 in, 1 out]
                      }
                    }
                  }
                  frame #1 {
                    n94 = flat-sequence {
                      tunnel: w335 -> [w345]
                      tunnel: w336 -> [w339]
                      frame #0 {
                        n95 = call "ESP300Write.vi"("error in (no error)"=errorcluster {"status"=FALSE, "code"=0, "source"=""}, "Command"="AG?", "ESP300 Axis"=w345, "ESP300 Address"=w339) -> ("error out"=w340:errorcluster)  [unwired: 3 in]
                        n96 = GPIB Read(0:w339, 1:64 ("byte count"), 3:w340, 4:300 ("timeout ms (488.2 global)")) -> (5:w343:string)  [unwired: 1 in, 2 out]
                        n97 = Fract/Exp String To Number(string=w343) -> (number=→"Current deceleration":dbl)  [unwired: 3 in, 1 out]
                      }
                    }
                  }
                }
              }
              frame True {
                n98 = stacked-sequence {
                  seq-local: [w350 _] -> [_ w361]
                  tunnel: w347 -> [w352 w363]
                  tunnel: w348 -> [w351 w362]
                  tunnel: errorcluster {"status"=FALSE, "code"=0, "source"=""} ("error in (no error)") -> [w349 w360]
                  frame #0 {
                    n99 = flat-sequence {
                      tunnel: w351 -> [w359]
                      tunnel: w352 -> [w355]
                      tunnel: ["Acceleration"] -> w350
                      tunnel: w349 -> [w353]
                      frame #0 {
                        n100 = Number To Fractional String(number="Acceleration") -> (F-format string=w358:string)  [unwired: 3 in]
                        n101 = Concatenate Strings("AC" ("string"), w358) -> (w356:string)
                        n102 = call "ESP300Write.vi"("error in (no error)"=w353, "Command"=w356, "ESP300 Axis"=w359, "ESP300 Address"=w355) -> ()  [unwired: 3 in, 1 out]
                      }
                    }
                  }
                  frame #1 {
                    n103 = flat-sequence {
                      tunnel: w362 -> [w370]
                      tunnel: w363 -> [w366]
                      tunnel: w361 -> [w365]
                      tunnel: w360 -> [w364]
                      frame #0 {
                        n104 = Number To Fractional String(number=w365) -> (F-format string=w369:string)  [unwired: 3 in]
                        n105 = Concatenate Strings("AG" ("string"), w369) -> (w367:string)
                        n106 = call "ESP300Write.vi"("error in (no error)"=w364, "Command"=w367, "ESP300 Axis"=w370, "ESP300 Address"=w366) -> ()  [unwired: 3 in, 1 out]
                      }
                    }
                  }
                }
              }
            }
          }
          frame #3 {
            # "Data Type Select"
            n107 = case shown="\"X\", 기본" "Enum" {
              tunnel: ["outp ? 1" "outp ? 2" "outp ? 3"] -> w372
              frame "X", Default {
              }
              frame "Y" {
              }
              frame "Abs" {
              }
            }
            "Data Type" <- w372
          }
          frame #4 {
            # "시뮬레이션용\n부울 함수"
            n108 = case shown="참" TRUE {
              tunnel: [w379 w381] -> w378
              tunnel: w376 -> [_ w380]
              frame False {
                n109 = Random Number (0-1)() -> (number: 0 to 1=w379:dbl)
              }
              frame True {
                n110 = call "readdata_830.vi"("Command"="outp ? 1", "timeout"=200, "Lockin Address"=w380) -> ("Data"=w381:dbl)  [unwired: 1 in, 1 out]
              }
            }
            "Lock-in X-Channel" <- w378
          }
          frame #5 {
            n111 = case shown="참" TRUE {
              tunnel: w385 -> [_ w389]
              tunnel: [w387 w388] -> w384
              frame False {
                n112 = Random Number (0-1)() -> (number: 0 to 1=w387:dbl)
              }
              frame True {
                n113 = call "readdata_830.vi"("Command"="outp ? 2", "timeout"=200, "Lockin Address"=w389) -> ("Data"=w388:dbl)  [unwired: 1 in, 1 out]
              }
            }
            "Lock-in Y-Channel" <- w384
          }
          frame #6 {
            n114 = case shown="거짓" "Reset Range" {
              frame False {
              }
              frame True {
                n115 = property on="Start Position" class="DigNum (엄격한)"() -> ("Value"=w394:sgl)  [unwired: 2 in, 2 out]
                n116 = property on="End Postion" class="DigNum (엄격한)"() -> ("Value"=w393:sgl)  [unwired: 2 in, 2 out]
                n117 = property on="THz Time-domain Signal Wave" class="XYGraph (엄격한)"("X Scale.Range:Minimum"=w394, "X Scale.Range:Maximum"=w393) -> ()  [unwired: 2 in, 2 out]
              }
            }
          }
        }
        n118 = Wait (ms)(milliseconds to wait=u32 150) -> ()  [unwired: 1 out]
      }
    }
    n119 = case shown="거짓" "Find Max" {
      tunnel: w36 -> [w65 _]
      tunnel: w35 -> [w64 _]
      frame True {
        n120 = call "FindMaxMin.vi"("x-axis"=w65, "y-axis"=w64) -> ("MaxPosition"=→"MaxPosition":dbl, "MaxValue"=→"MaxValue":dbl, "MinPosition"=→"MinPosition":dbl, "MinValue"=→"MinValue":dbl)
      }
      frame False {
      }
    }
    n121 = case shown="거짓" "Save Data" {
      tunnel: w36 -> [w46 w59]
      tunnel: w35 -> [w47 w58]
      tunnel: [w49 w59] -> w38
      tunnel: [w48 w58] -> w37
      frame True {
        n122 = stacked-sequence {
          tunnel: w47 -> [w51]
          tunnel: w46 -> [w52]
          tunnel: [w52] -> w49
          tunnel: [w51] -> w48
          frame #0 {
            n123 = Divide(x=w52, y=sgl 0.15) -> (x/y=w53:sgl[])
            n124 = Build Array (concatenate)(w53, w51) -> (w50:dbl[])
            n125 = call-poly <vilib>:"Write To Spreadsheet File.vi"("transpose? (no:F)"=TRUE ("transpose?\n(no:F)"), "format (%.3f)"="%.6e", "append to file? (new file:F)"=FALSE ("append to file?\n(new file:F)"), "1D data"=w50) -> ()  [unwired: 4 in, 1 out]
          }
        }
      }
      frame False {
      }
    }
    n126 = Unbundle(w28) -> ("System no."=w27:i32, "error out"=w26:errorcluster)
  }
  n127 = call "ERR?.vi"("error in"=w1) -> ("error out"=w4:errorcluster)  [unwired: 17 in, 1 out]
  n128 = call "GCSTranslateError.vi"("error in"=w4) -> ("error out"=w3:errorcluster)  [unwired: 16 in, 2 out]
  n129 = call "Close connection if open.vi"("System no."=w2, "error in"=w3) -> ("error out"=→"error out":errorcluster)  [unwired: 16 in, 1 out]
